vi "To Generic.vi"(8 "error in (no error)":errorcluster, 11 "Request Data in":refnum<class "Tracker Data.lvclass">) -> (0 "error out":errorcluster, 2 "Generic Data":refnum<class "Generic Data.lvclass">[](array[class]), 3 "Data Name":string[](array[string]))   [LabVIEW 2020, in "Data Tracker.lvlib" / "Tracker Data.lvclass"]
doc: "Present private data as an array of named generic data elements."
uses:
  Tracker Data.lvclass
  PPL/HDH.Data.Generic.lvlibp/Generic Data/Generic Data.lvclass
  Tracker Data.lvclass/Tracker Data.ctl
  PPL/HDH.Data.Generic.lvlibp/Generic Data/U32/U32.lvclass
  C:/Current projects/WS/PPL/HDH.Data.Generic.lvlibp/Generic Data/Generic Data.lvclass
  PPL/HDH.Actor Framework.Core.Publisher.lvlibp/Messages/Timed Msg/Data/Timed Data/Timed Data.lvclass
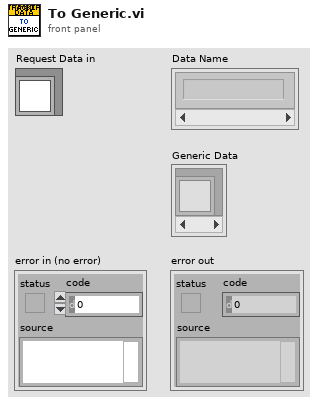
[diagram p1: front panel]
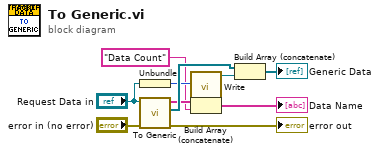
[diagram p0: block diagram]
diagram:
  n1 = Unbundle("Request Data in") -> (w7:u32)
  n2 = call-parent "To Generic.vi"("error in (no error)"="error in (no error)", "Request Data in"="Request Data in") -> ("error out"=→"error out":errorcluster, "Generic Data"=w10:refnum<class "Generic Data.lvclass">[], "Data Name"=w4:string[])  [unwired: 7 in]
  n3 = call "Write.vi"("U32"=w7) -> ("U32 out"=w5:refnum<class "U32.lvclass">)  [unwired: 10 in]
  n4 = Build Array (concatenate)(w4, "Data Count" ("element")) -> (→"Data Name":string[])
  n5 = Build Array (concatenate)(w10, w5) -> (→"Generic Data":refnum<class "Generic Data.lvclass">[])
